vi "Set Mode.vi"(8 "error in (no error)":errorcluster, 10 "Mode":T1, 11 "Stream in":refnum<class "Stream.lvclass">) -> (0 "error out":errorcluster, 3 "Stream out":refnum<class "Stream.lvclass">)   [LabVIEW 2020, in "Stream.lvlib" / "Stream.lvclass"]
uses:
  Stream.lvclass
  Mode.ctl
  Stream.lvclass/Stream.ctl
  Stream.lvlib
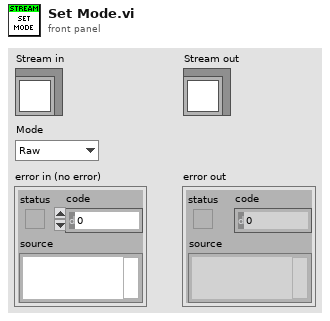
[diagram p1: front panel]
types:
  T1 = typedef "Stream.lvlib/Mode.ctl" = enum16{"Raw", "Buffered", "LineTerm"}
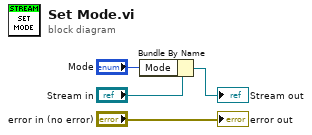
[diagram p0: block diagram]
diagram:
  n1 = Bundle By Name(cluster="Stream in", "Mode"="Mode") -> (→"Stream out":refnum<class "Stream.lvclass">)
  "error out" <- "error in (no error)"
